vi "Check for Command.vi"(10 "Check Only":bool, 11 "Array":string[](array[string])) -> (2 "Argument Out":string, 3 "Array Out":string[](array[string]), 5 "Found Out":bool)   [LabVIEW 2020]
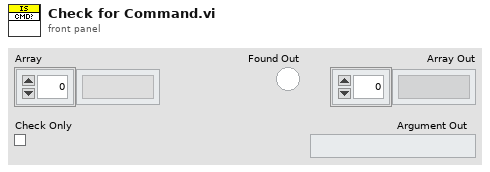
[diagram p1: front panel]
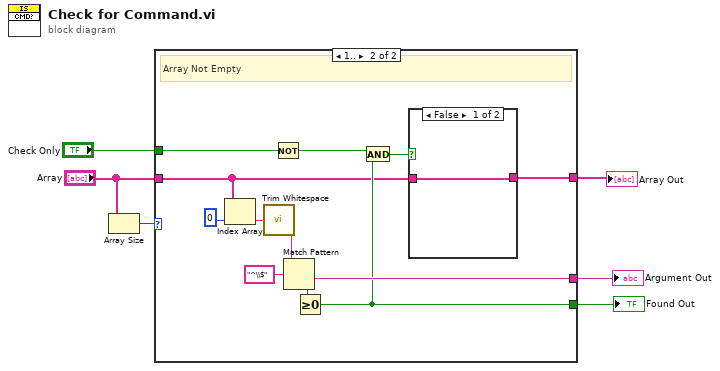
[diagram p0: block diagram]
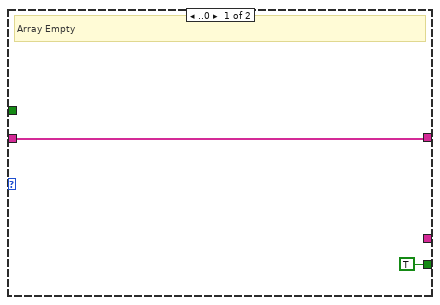
[diagram p2: hidden frame]
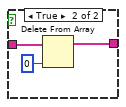
[diagram p3: hidden frame]
diagram:
  n1 = Array Size(array="Array") -> (size(s)=w1:i32)
  n2 = case shown="1.." w1 {
    tunnel: [_ w20] -> w6
    tunnel: [TRUE w13] -> w5
    tunnel: "Check Only" -> [_ w12]
    tunnel: [w7 w10] -> w3
    tunnel: "Array" -> [w7 w9]
    frame ..0 {
      # "Array Empty"
    }
    frame 1.. {
      # "Array Not Empty"
      n3 = Index Array(array=w9, index=0) -> (element=w16:string)
      n4 = call <vilib>:"Trim Whitespace.vi"("string"=w16) -> ("trimmed string"=w18:string)  [unwired: 1 in]
      n5 = Not(x=w12) -> (.not. x?=w11:bool)
      n6 = Match Pattern(string=w18, regular expression="^\\$") -> (after substring=w20:string, offset past match=w19:i32)  [unwired: 1 in, 2 out]
      n7 = Greater Or Equal To 0?(x=w19) -> (x >= 0?=w13:bool)
      n8 = And(x=w11, y=w13) -> (x .and. y?=w14:bool)
      n9 = case shown="False" w14 {
        tunnel: w9 -> [w21 w24]
        tunnel: [w21 w23] -> w10
        frame False {
        }
        frame True {
          n10 = Delete From Array(array=w24, index=0) -> (array with subset deleted=w23:string[])  [unwired: 1 in, 1 out]
        }
      }
    }
  }
  "Argument Out" <- w6
  "Found Out" <- w5
  "Array Out" <- w3
